vi "ctx estimate now sync value v2.vi"(11 "context":u32) -> (2 "function return":u64, 3 "context out":u32)   [LabVIEW 2019, in "apdm.lvlib"]
doc: "APDM_EXPORT uint64_t apdm_ctx_estimate_now_sync_value_v2(apdm_ctx_t context);"
uses:
  apdm.lvlib
  Lee Lab/CP FES Walking 2018/Code/Working/LabVIEW/apdm.dll
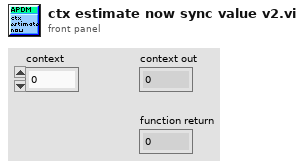
[diagram p1: front panel]
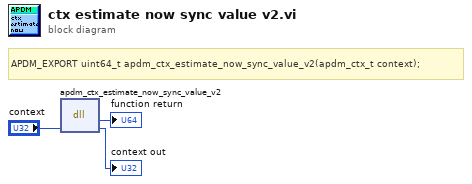
[diagram p0: block diagram]
diagram:
  # "APDM_EXPORT uint64_t apdm_ctx_estimate_now_sync_value_v2(apdm_ctx_t context);"
  n1 = dll-call lib="C:/Users/jfalesi/Dropbox/Lee Lab/CP FES Walking 2018/Code/Working/LabVIEW/apdm.*" fn="apdm_ctx_estimate_now_sync_value_v2"("context"="context") -> (→"function return":u64, "context"=→"context out":u32)  [unwired: 3 in, 2 out]
